vi "User access global.vi"(8 "error in (no error)":errorcluster, 9 "Set Loged in":bool, 10 "User access set":T1 {"Expire sec" format="%.2f"}, 11 "Set? (get)":bool) -> (0 "error out":errorcluster, 1 "Administrator":bool, 2 "User access":T1 {"Expire sec" format="%.2f"}, 3 "Valid user loged in?":bool, 5 "User ID":string)   [LabVIEW 2013]
uses:
  User Access Type defs/User access cluster.ctl
  User Access Type defs/Security level U8.ctl
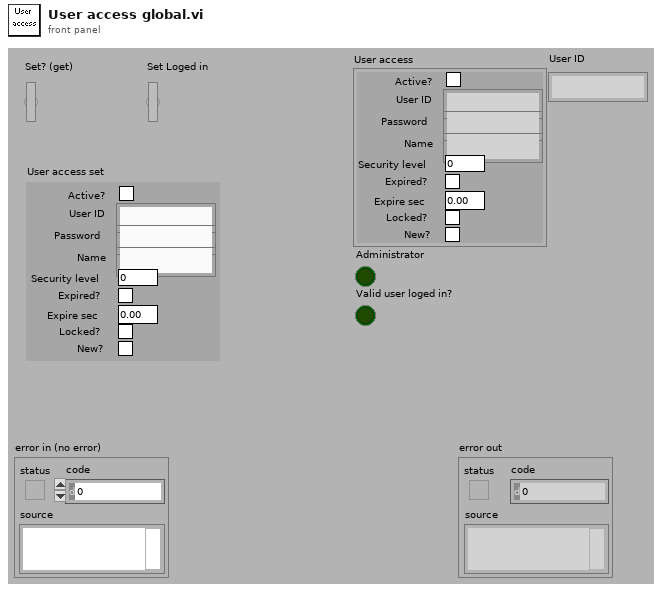
[diagram p1: front panel]
types:
  T1 = typedef "User access cluster.ctl" = cluster{"Active?":bool, "User ID":string, "Password":string, "Name":string, "Security level":T2, "Expired?":bool, "Expire sec":dbl, "Locked?":bool, "New?":bool}
  T2 = typedef "Security level U8.ctl" = u8
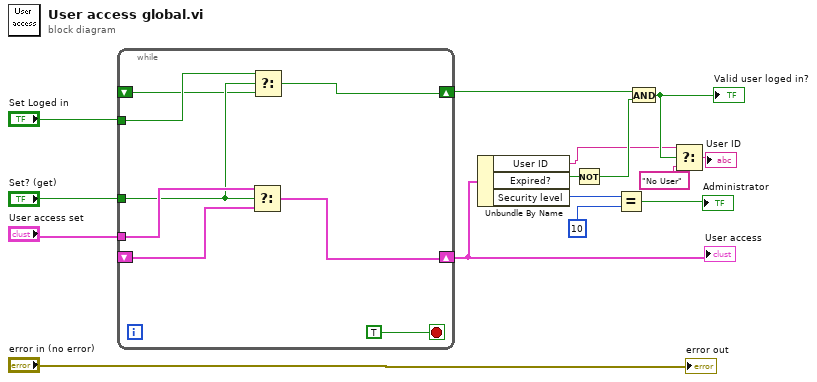
[diagram p0: block diagram]
diagram:
  n1 = while {
    shift-right: [w22] -> w13
    shift-left: _ -> [w20]
    tunnel: "Set? (get)" -> [w19]
    tunnel: "User access set" -> [w21]
    shift-right: [w16] -> w7
    shift-left: _ -> [w17]
    tunnel: "Set Loged in" -> [w18]
    stop <- TRUE ("stop") stop-if-true
    n2 = Select(t=w21, s=w19, f=w20) -> (s? t:f=w22:T1)
    n3 = Select(t=w18, s=w19, f=w17) -> (s? t:f=w16:bool)
  }
  "User access" <- w13
  n4 = Unbundle By Name(w13) -> ("User ID"=w3:string, "Expired?"=w6:bool, "Security level"=w11:T2)
  n5 = Not(x=w6) -> (.not. x?=w5:bool)
  n6 = Equal?(x=w11, y=T2 10) -> (x = y?=→"Administrator":bool)
  n7 = And(x=w7, y=w5) -> (x .and. y?=w4:bool)
  "Valid user loged in?" <- w4
  n8 = Select(t=w3, s=w4, f="No User") -> (s? t:f=→"User ID":string)
  "error out" <- "error in (no error)"
